vi "nominal debug open handles.vi"(8 "error in (no error)":errorcluster, 9 "out_needed":u32, 10 "cap":u32, 11 "buf":string) -> (0 "error out":errorcluster, 1 "out_needed out":u32, 2 "function return":i32, 3 "buf out":string)   [LabVIEW 2020, in "client.lvlib"]
doc: "int32_t nominal_debug_open_handles(char *buf, uint32_t cap, uint32_t *out_needed);"
uses:
  client.lvlib
  bin/nominalClient_64.dll
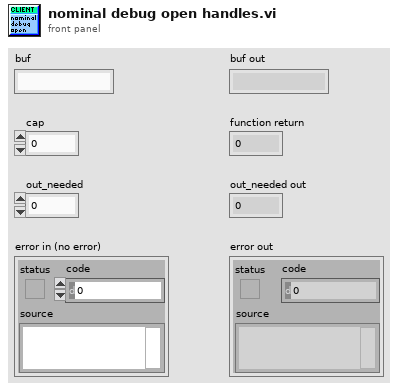
[diagram p1: front panel]
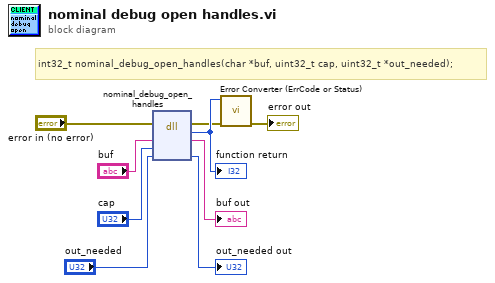
[diagram p0: block diagram]
diagram:
  # "int32_t nominal_debug_open_handles(char *buf, uint32_t cap, uint32_t *out_needed);"
  n1 = dll-call lib="C:/code/labview-client-rs/lv_src/bin/nominalClient_*.*" fn="nominal_debug_open_handles"(error in="error in (no error)", "buf"="buf", "cap"="cap", "out_needed"="out_needed") -> (error out=w2:errorcluster, w9:i32, "buf"=→"buf out":string, "out_needed"=→"out_needed out":u32)  [unwired: 3 in, 1 out]
  "function return" <- w9
  n2 = call "Error Converter (ErrCode or Status).vi"("error in (no error)"=w2, "error code"=w9) -> ("error out"=→"error out":errorcluster)  [unwired: 9 in]
